vi "niFPGALMRsmpl1MInSCTL.vi"(0 "input data":fxp<+/-,16,16>, 1 "reset":bool, 9 "input valid":bool=TRUE, 12 "ready for output":bool=TRUE) -> (3 "channel index":u8, 4 "output data":fxp<+/-,18,1>, 10 "output valid":bool, 14 "ready for input":bool=TRUE)   [LabVIEW 2017]
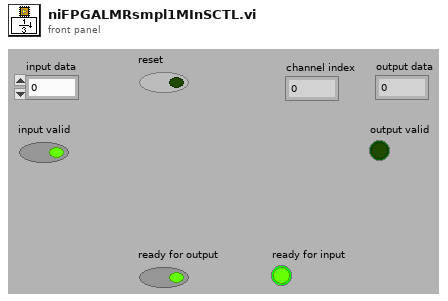
[diagram p1: front panel]
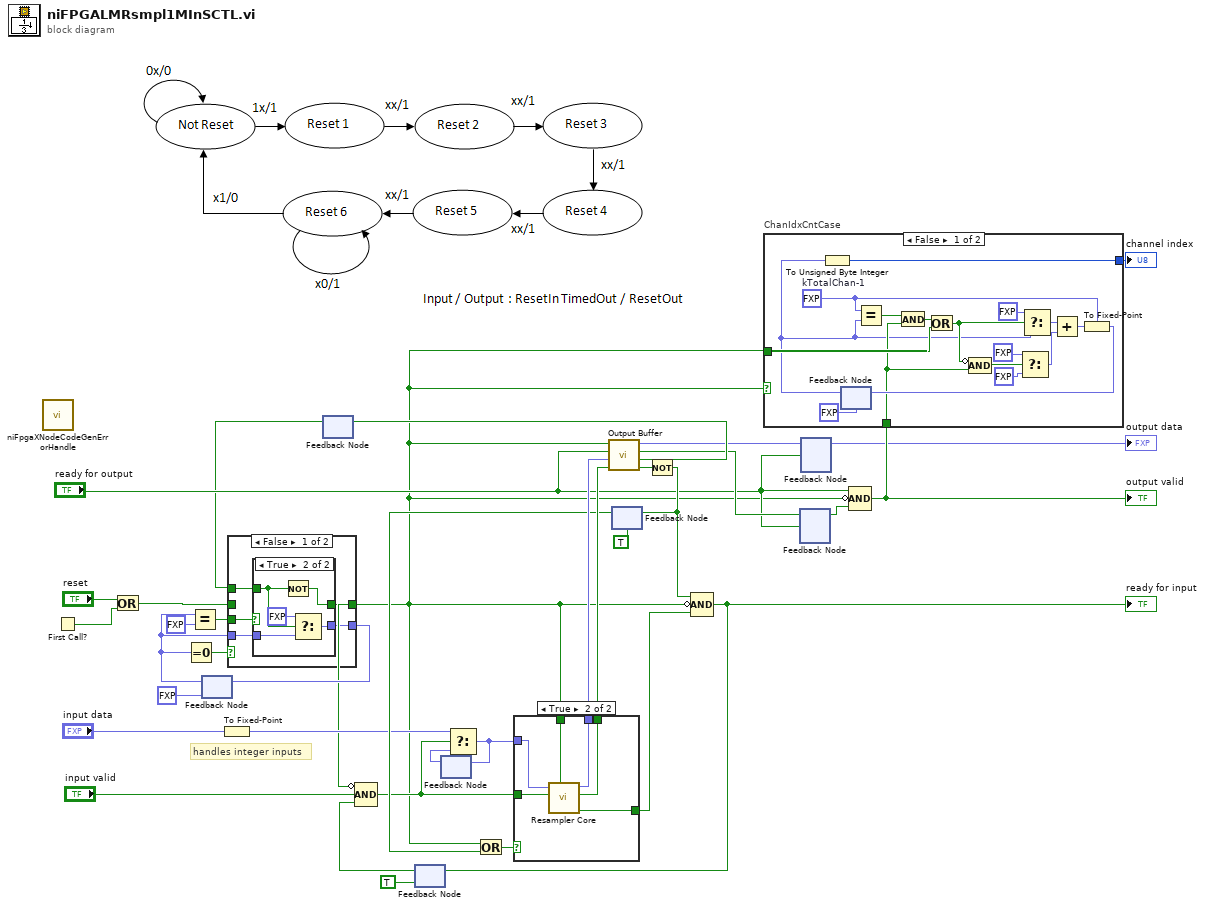
[diagram p0: block diagram]
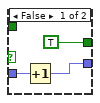
[diagram p2: hidden frame]
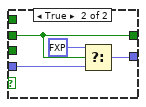
[diagram p3: hidden frame]
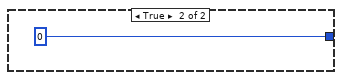
[diagram p4: hidden frame]
diagram:
  # "handles integer inputs"
  n1 = call <vilib>:"niFpgaXNodeCodeGenErrorHandle.vi"() -> ()  [unwired: 1 in]
  n2 = First Call?() -> (First Call?: T/F=w30:bool)
  n3 = Or(x="reset", y=w30) -> (x .or. y?=w2:bool)
  n4 = feedback #1(fxp<+,3,3> 0.0) -> (w7:fxp<+,3,3>)
  n5 = Equal To 0?(x=w7) -> (x = 0?=w8:bool)
  n6 = Equal?(x=w7, y=fxp<+,3,3> 6.0) -> (x = y?=w5:bool)
  n7 = To Fixed-Point(number="input data") -> (fixed-point=w10:fxp<+/-,16,16>)  [unwired: 1 in]
  n8 = feedback #2() -> (w1:bool)  [unwired: 1 out]
  n9 = case shown="False" w8 {
    tunnel: w2 -> [_ w52]
    tunnel: [w38 w53] -> w4
    tunnel: [w40 w52] -> w3
    tunnel: w7 -> [w39 w51]
    tunnel: w5 -> [w41 _]
    tunnel: w1 -> [w37 _]
    frame False {
      n10 = case shown="True" w41 {
        tunnel: [TRUE w49] -> w40
        tunnel: w39 -> [w43 w45]
        tunnel: [w42 w48] -> w38
        tunnel: w37 -> [_ w47]
        frame False {
          n11 = Increment(x=w43) -> (x+1=w42:fxp<+,3,3>)
        }
        frame True {
          n12 = Not(x=w47) -> (.not. x?=w49:bool)
          n13 = Select(t=fxp<+,3,3> 0.0, s=w47, f=w45) -> (s? t:f=w48:fxp<+,3,3>)
        }
      }
    }
    frame True {
      n14 = Select(t=fxp<+,3,3> 1.0, s=w52, f=w51) -> (s? t:f=w53:fxp<+,3,3>)
    }
  }
  n15 = feedback-in #1(w4) -> ()
  n16 = feedback #3(TRUE) -> (w34:bool)
  n17 = Compound Arithmetic op=AND(invert w3, "input valid", w34) -> (w17:bool)
  n18 = feedback #4() -> (w26:fxp<+/-,16,16>)  [unwired: 1 out]
  n19 = Select(t=w10, s=w17, f=w26) -> (s? t:f=w25:fxp<+/-,16,16>)
  n20 = feedback-in #4(w25) -> ()
  n21 = feedback #5(TRUE) -> (w20:bool)
  n22 = Or(x=w3, y=w20) -> (x .or. y?=w33:bool)
  n23 = case "MultiRateFilterEnableCaseStructure_xxx" shown="True" w33 {
    tunnel: w17 -> [_ w57]
    tunnel: w3 -> [_ w58]
    tunnel: [_ w56] -> w28
    tunnel: [_ w55] -> w27
    tunnel: [_ w59] -> w32
    tunnel: w25 -> [_ w54]
    frame False {
    }
    frame True {
      n24 = call "Resampler Core"("reset"=w58, "dataRDYIn"=w57, "datain"=w54) -> ("idle?"=w59:bool, "dataReadyOut"=w55:bool, "output data"=w56:fxp<+/-,18,1>)  [unwired: 6 in]
    }
  }
  n25 = call "Output Buffer"("wrEn"=w27, "wrVal"=w28, "ready for output"="ready for output", "reset"=w3) -> ("wrTimedOut?"=w19:bool, "rdTimedOut?"=w29:bool, "outputValid"=w13:bool, "outputData"=w15:fxp<+/-,18,1>)  [unwired: 4 in]
  n26 = feedback-in #2(w29) -> ()
  n27 = Not(x=w19) -> (.not. x?=w16:bool)
  n28 = feedback-in #5(w16) -> ()
  n29 = Compound Arithmetic op=AND(w16, invert w3, w32) -> (w35:bool)
  "ready for input" <- w35
  n30 = feedback-in #3(w35) -> ()
  n31 = feedback #6() -> (w11:bool)  [unwired: 1 in]
  n32 = feedback-in #6(w13, "ready for output") -> ()
  n33 = feedback #7() -> (→"output data":fxp<+/-,18,1>)  [unwired: 1 in]
  n34 = feedback-in #7(w15, "ready for output") -> ()
  n35 = Compound Arithmetic op=AND("ready for output", invert w3, w11) -> (w22:bool)
  "output valid" <- w22
  n36 = case "ChanIdxCntCase" shown="False" w3 {
    tunnel: w3 -> [w63 _]
    tunnel: w22 -> [w62 _]
    tunnel: [w76 u8 0] -> w21
    frame False {
      w64 = fxp<+,1,1> 0.0  # kTotalChan-1
      n37 = feedback #8(fxp<+,1,1> 0.0) -> (w61:fxp<+,1,1>)
      n38 = To Unsigned Byte Integer(number=w61) -> (unsigned 8bit integer=w76:u8)
      n39 = Equal?(x=w64, y=w61) -> (x = y?=w75:bool)
      n40 = And(x=w75, y=w62) -> (x .and. y?=w74:bool)
      n41 = Or(x=w74, y=w63) -> (x .or. y?=w73:bool)
      n42 = Compound Arithmetic op=AND(invert w73, w62) -> (w70:bool)
      n43 = Select(t=fxp<+,1,1> 1.0 ("y"), s=w70, f=fxp<+,1,1> 0.0) -> (s? t:f=w67:fxp<+,1,1>)
      n44 = Select(t=fxp<+,1,1> 0.0 ("y"), s=w73, f=w61) -> (s? t:f=w71:fxp<+,1,1>)
      n45 = Add(x=w71, y=w67) -> (x+y=w66:fxp<+,2,2>)
      n46 = To Fixed-Point(fixed-point type=w64, number=w66) -> (fixed-point=w65:fxp<+,1,1>)
      n47 = feedback-in #8(w65) -> ()
    }
    frame True {
    }
  }
  "channel index" <- w21
